vi "commutation.vi"(8 "error in (no error)":errorcluster, 10 "Theta [deg] Array In":dbl[](array[numeric]), 11 "Torque Cmd - Td [Ncm]":dbl) -> (0 "error out":errorcluster, 1 "Voltage 2 [V]":dbl, 2 "Voltage 1 [V]":dbl)   [LabVIEW 2018]
doc: "For a given torque command and the angles of motor 1 and motor 2, runs the commutation algorithm which minimizes the total power consumption and outputs voltage-1, voltage-2 for each motor to provide the net torque."
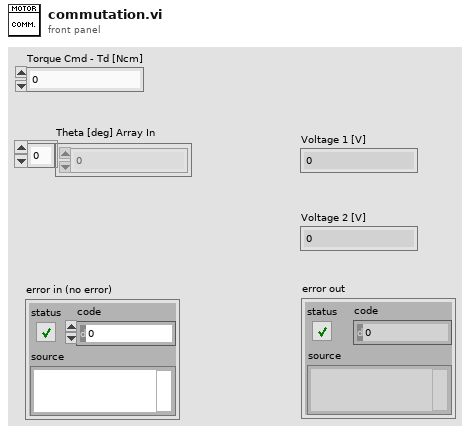
[diagram p1: front panel]
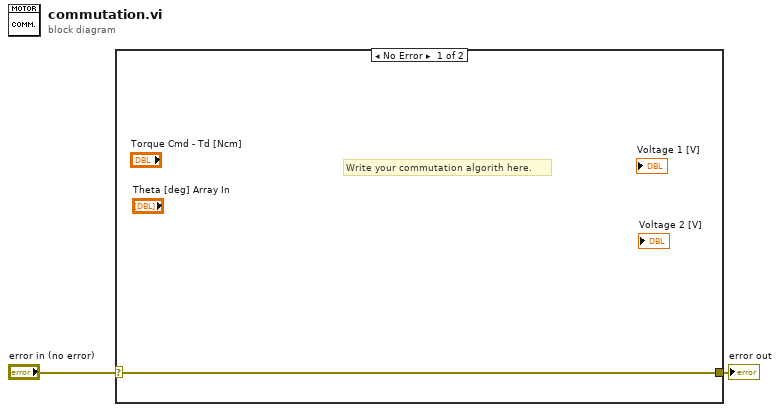
[diagram p0: block diagram]
diagram:
  n1 = case shown="No Error" "error in (no error)" {
    selector: "error in (no error)" -> [w3 w4]
    tunnel: [w3 w4] -> w1
    frame No Error {
      # "Write your commutation algorith here."
    }
    frame Error {
    }
  }
  "error out" <- w1
